vi "Autonomous.vi"   [LabVIEW 2020]
doc: "This VI starts when autonomous period begins, and will automatically be terminated when it ends. You can carry out timed or sensor driven operations directly to I/O or to subsystems without needing to return to the caller."
uses:
  Swerve/Implementation/Swerve Setpoints.ctl
  Swerve/Implementation/Swerve Operations.ctl
  <vilib>/Rock Robotics/WPI/Framework/Completion Status.ctl
  <vilib>/Rock Robotics/WPI/Utilities/WPI_GetSetVariantRefNum.vi
  <vilib>/Rock Robotics/Network Tables/NT Read String.vi
types:
  T1 = typedef "WPI_JoystickDevRef.ctl" = cluster{"Device":T2}
  T2 = typedef "WPI_JoystickDeviceEnum.ctl" = enum16{"USB 0", "USB 1", "USB 2", "USB 3", "USB 4", "USB 5"}
  T3 = typedef "Swerve Operations.ctl" = enum16{"Reserve", "Read Current", "Immediate", "Joystick Drive", "Drive for Time", "Turn to Angle", "Drive to Angle(Time)", "Drive for Distance", "Drive to Angle(Distance)"}
  T4 = typedef "Swerve Setpoints.ctl" = cluster{"Operation":T3, "Gyro":dbl, "Rotate":dbl, "Time":dbl, "Foward":dbl, "Distance":dbl, "Strafe":dbl, "Right Trigger":dbl, "Angle":dbl, "Start Angle":dbl}
  T5 = typedef "Completion Status.ctl" = enum16{"Successful", "Aborted", "Incomplete"}
  T6 = typedef "WPI_MotorControlDeviceRef.ctl" = cluster{"DeviceStatus":errorcluster, "Type":T7, "PWM":cluster{"PWM Channel":T8, "DeadBand":T9}, "CAN":cluster{"Device Number":u8, "SetOutput VI Ref":variant, "GetOutput VI Ref":variant, "Enable VI Ref":variant, "Disable VI Ref":variant, "Data":variant}, "Invert":bool, "DIO PWM":cluster{"PWM \"Enable\" Channel":T8, "DIOChannel":T10, "PWM Rate":dbl}}
  T7 = typedef "WPI_MotorControlType.ctl" = enum16{"PWM", "CAN", "DIO PWM"}
  T8 = typedef "FPGA_DIOPWMChannel.ctl" = enum8{"PWM 0", "PWM 1", "PWM 2", "PWM 3", "PWM 4", "PWM 5", "PWM 6", "PWM 7", "PWM 8", "PWM 9", "PWM MXP 0", "PWM MXP 1", "PWM MXP 2", "PWM MXP 3", "PWM MXP 4", "PWM MXP 5", "PWM MXP 6", "PWM MXP 7", "PWM MXP 8", "PWM MXP 9", "Invalid"}
  T9 = typedef "WPI_PWMDeadband.ctl" = cluster{"Name":string, "maxPositivePwm":i32, "minPositivePwm":i32, "centerPwm":i32, "maxNegativePwm":i32, "minNegativePwm":i32, "angularRange":u16}
  T10 = typedef "FPGA_DIOChannel.ctl" = enum8{"DIO 0", "DIO 1", "DIO 2", "DIO 3", "DIO 4", "DIO 5", "DIO 6", "DIO 7", "DIO 8", "DIO 9", "DIO MXP 0", "DIO MXP 1", "DIO MXP 2", "DIO MXP 3", "DIO MXP 4", "DIO MXP 5", "DIO MXP 6", "DIO MXP 7", "DIO MXP 8", "DIO MXP 9", "DIO MXP 10", "DIO MXP 11", "DIO MXP 12", "DIO MXP 13", "DIO MXP 14", "DIO MXP 15", "SPI Port CS1", "SPI Port CS2", "SPI Port CS3", "SPI Port MISO", "SPI Port MOSI", "Invalid"}
  T11 = typedef "ADIS16470 Device Reference.ctl" = cluster{"DevStatus":errorcluster, "Hardware Config":T12, "Calibration Complete":refnum<notifier>, "Status Reference":refnum<data-value>, "Data Reference":refnum<data-value>, "Sychronous Process VI":T15, "Cmd FIFO":refnum<k33>, "Source":T16, "Data FIFO":refnum<k33>, "Calibration Time (ms)":u32, "Data Reference":refnum<data-value>}
  T12 = typedef "ADIS16470 Hardware Configuration.ctl" = cluster{"SPI Clock Rate (Hz)":dbl, "IMU SPI Mode (3)":T13, "IMU Reset Pin":T10, "IMU SPI Bus":T14, "IMU Data Ready Pin":T10, "Stall Config":cluster{"Pow2BytesPerRead":u8, "StallTicks":u16, "CsToSclkTicks":u8}}
  T13 = typedef "WPI_SPIMode.ctl" = enum16{"Mode 0 (Clk Idle Low,Sample on Leading)", "Mode 1 (Clk Idle Low,Sample on Trailing)", "Mode 2 (Clk Idle High,Sample on Leading)", "Mode 3 (Clk Idle High,Sample on Trailing)"}
  T14 = typedef "spi_bus.ctl" = enum16{"SPI On-Board, CS0", "SPI On-Board, CS1", "SPI On-Board, CS2", "SPI On-Board, CS3", "SPI MXP", "Invalid"}
  T15 = typedef "ADIS16470 Process.ctl" = refnum<vi>
  T16 = typedef "FPGA_CounterEncoderSourceConvertionLVSourceType.ctl" = cluster{"DevStatus":errorcluster, "AnalogTriggerMode?":bool, "DigitalMode":cluster{"DIO Channel":T17}, "AnalogTriggerMode":cluster{"AnalogTriggerIndex":T18, "OutputType":T19}}
  T17 = typedef "FPGA_DIODigitalSourceChannel.ctl" = enum8{"DIO 0", "DIO 1", "DIO 2", "DIO 3", "DIO 4", "DIO 5", "DIO 6", "DIO 7", "DIO 8", "DIO 9", "DIO MXP 0", "DIO MXP 1", "DIO MXP 2", "DIO MXP 3", "DIO MXP 4", "DIO MXP 5", "DIO MXP 6", "DIO MXP 7", "DIO MXP 8", "DIO MXP 9", "DIO MXP 10", "DIO MXP 11", "DIO MXP 12", "DIO MXP 13", "DIO MXP 14", "DIO MXP 15", "SPI Port CS1", "SPI Port CS2", "SPI Port CS3", "SPI Port MISO", "SPI Port MOSI", "Disabled"}
  T18 = typedef "FPGA_AnalogTriggerIndex.ctl" = enum8{"Trig 0", "Trig 1", "Trig 2", "Trig 3", "Trig 4", "Trig 5", "Trig 6", "Trig 7", "Invalid"}
  T19 = typedef "FPGA_AnalogTriggerOutType.ctl" = enum16{"InWindow", "TriggerState", "Rising", "Falling"}
  T20 = typedef "ADIS16470 Data.ctl" = cluster{"XAngle":dbl, "YAngle":dbl, "ZAngle":dbl}
  T21 = typedef "Command Status Info.ctl" = cluster{"Name":string, "Status":T5, "notifier out":T22}
  T22 = typedef "Completion Notifier.ctl" = refnum<notifier>
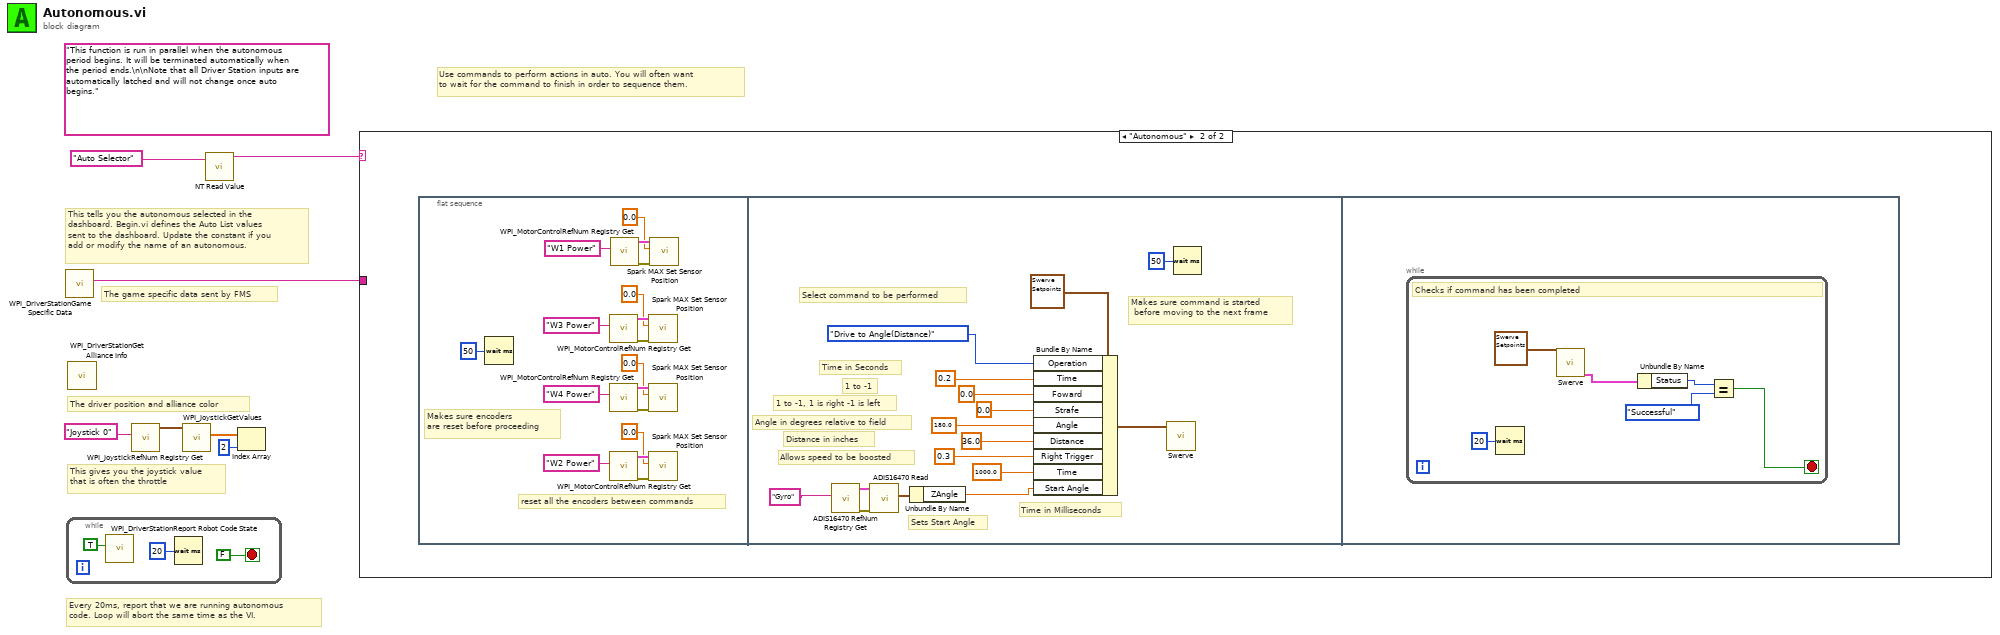
[diagram p0: block diagram]
diagram:
  (unwired) "This function is run in parallel when the autonomous period begins. It will be terminated automatically when the period ends.\n\nNote that all Driver Station inputs are automatically latched and will not change once auto begins."
  # "The game specific data sent by FMS"
  # "This tells you the autonomous selected in the \ndashboard. Begin.vi defines the Auto List values\nsent to the dashboard. Update the constant if you\nadd or modify the name of an autonomous."
  # "Every 20ms, report that we are running autonomous\ncode. Loop will abort the same time as the VI."
  # "This gives you the joystick value\nthat is often the throttle"
  # "Use commands to perform actions in auto. You will often want\nto wait for the command to finish in order to sequence them."
  # "The driver position and alliance color"
  n1 = call <vilib>:"WPI_DriverStationGame Specific Data.vi"() -> ("Game Specific Data"=w1:string)  [unwired: 11 in]
  n2 = while {
    stop <- FALSE stop-if-true
    n3 = call <vilib>:"WPI_DriverStationReport Robot Code State.vi"("Autonomous"=TRUE) -> ()  [unwired: 10 in, 1 out]
    n4 = Wait (ms)(milliseconds to wait=u32 20) -> ()  [unwired: 1 out]
  }
  n5 = call <vilib>:"WPI_DriverStationGet Alliance Info.vi"() -> ()  [unwired: 12 out]
  n6 = call <vilib>:"WPI_JoystickRefNum Registry Get.vi"("refnum name"="Joystick 0") -> ("JoystickDevRef"=w6:T1)  [unwired: 1 in, 9 out]
  n7 = call <vilib>:"WPI_JoystickGetValues.vi"("JoystickDevRef"=w6) -> ("Axes"=w5:dbl[])  [unwired: 6 in, 4 out]
  n8 = call-poly <vilib>:"NT Read Value.vi"("Name"="Auto Selector") -> ("String"=w2:string)  [unwired: 9 in, 1 out]
  n9 = Index Array(array=w5, index=2) -> ()  [unwired: 1 out]
  n10 = case shown="\"Autonomous\"" w2 {
    tunnel: w1 -> [_ _]
    frame Default {
      # "You can put your main auto here, or you can right-click on the case and make any\nother frame be the default case."
      # "This is the frame that will execute if no selection is made, or if it is not recognized"
    }
    frame "Autonomous" {
      n11 = flat-sequence {
        frame #0 {
          # "Makes sure encoders \nare reset before proceeding"
          # "reset all the encoders between commands"
          n12 = Wait (ms)(milliseconds to wait=u32 50) -> ()  [unwired: 1 out]
          n13 = call <vilib>:"WPI_MotorControlRefNum Registry Get.vi"("refnum name"="W3 Power") -> ("error out"=w24:errorcluster, "MotorControlDevRef"=w25:T6)  [unwired: 9 in]
          n14 = call <vilib>:"WPI_MotorControlRefNum Registry Get.vi"("refnum name"="W4 Power") -> ("error out"=w26:errorcluster, "MotorControlDevRef"=w27:T6)  [unwired: 9 in]
          n15 = call <vilib>:"WPI_MotorControlRefNum Registry Get.vi"("refnum name"="W2 Power") -> ("error out"=w22:errorcluster, "MotorControlDevRef"=w23:T6)  [unwired: 9 in]
          n16 = call <vilib>:"WPI_MotorControlRefNum Registry Get.vi"("refnum name"="W1 Power") -> ("error out"=w20:errorcluster, "MotorControlDevRef"=w21:T6)  [unwired: 9 in]
          n17 = call <vilib>:"Spark MAX Set Sensor Position.vi"("error in"=w24, "Position"=0.0, "MotorControlDeviceRef"=w25) -> ()  [unwired: 7 in, 2 out]
          n18 = call <vilib>:"Spark MAX Set Sensor Position.vi"("error in"=w26, "Position"=0.0, "MotorControlDeviceRef"=w27) -> ()  [unwired: 7 in, 2 out]
          n19 = call <vilib>:"Spark MAX Set Sensor Position.vi"("error in"=w22, "Position"=0.0, "MotorControlDeviceRef"=w23) -> ()  [unwired: 7 in, 2 out]
          n20 = call <vilib>:"Spark MAX Set Sensor Position.vi"("error in"=w20, "Position"=0.0, "MotorControlDeviceRef"=w21) -> ()  [unwired: 7 in, 2 out]
        }
        frame #1 {
          # "Select command to be performed"
          # "1 to -1"
          # "1 to -1, 1 is right -1 is left"
          # "Angle in degrees relative to field"
          # "Time in Seconds"
          # "Distance in inches"
          # "Time in Milliseconds"
          # "Allows speed to be boosted"
          # "Sets Start Angle"
          # "Makes sure command is started\n before moving to the next frame"
          n21 = call <vilib>:"ADIS16470 RefNum Registry Get.vi"("refnum name"="Gyro") -> ("error out"=w43:errorcluster, "ADIS16470DevRef out"=w42:T11)  [unwired: 9 in]
          n22 = call <vilib>:"ADIS16470 Read.vi"("error in (no error)"=w43, "ADIS16470DevRef"=w42) -> ("ADIS16470 Value"=w41:T20)  [unwired: 6 in, 3 out]
          n23 = Unbundle By Name(w41) -> ("ZAngle"=w28:dbl)
          n24 = Bundle By Name(cluster=T4 {"Operation"=enum."Reserve", "Gyro"=0.0, "Rotate"=0.0, "Time"=0.0, "Foward"=0.0, "Distance"=0.0, "Strafe"=0.0, "Right Trigger"=0.0, "Angle"=0.0, "Start Angle"=0.0} ("SubSystem Data"), "Operation"=Swerve_Operations."Drive to Angle(Distance)", "Time"=0.2 ("FWD"), "Foward"=0.0 ("STR"), "Strafe"=0.0, "Angle"=180.0, "Distance"=36.0, "Right Trigger"=0.3, "Time"=1000.0, "Start Angle"=w28) -> (w36:T4)
          n25 = call "Swerve.vi"("SubSystem Data"=w36) -> ()  [unwired: 10 in, 1 out]
          n26 = Wait (ms)(milliseconds to wait=u32 50) -> ()  [unwired: 1 out]
        }
        frame #2 {
          n27 = while {
            stop <- w45 stop-if-true
            # "Checks if command has been completed"
            n28 = Wait (ms)(milliseconds to wait=u32 20) -> ()  [unwired: 1 out]
            n29 = call "Swerve.vi"("SubSystem Data"=T4 {"Operation"=enum."Read Current", "Gyro"=0.0, "Rotate"=0.0, "Time"=0.0, "Foward"=0.0, "Distance"=0.0, "Strafe"=0.0, "Right Trigger"=0.0, "Angle"=0.0, "Start Angle"=0.0}) -> ("Command Info Out"=w46:T21)  [unwired: 10 in]
            n30 = Unbundle By Name(w46) -> ("Status"=w47:T5)
            n31 = Equal?(x=w47, y=Completion_Status."Successful") -> (x = y?=w45:bool)
          }
        }
      }
    }
  }
